vi "SR1.get Number of Stored Data.vi"(0 "i ref in":refnum<vi>, 5 "error in (no error)":errorcluster) -> (14 "i ref out":refnum<vi>, 16 "NofStoredData":i32, 19 "error out":errorcluster)   [LabVIEW 2014, in "SR1.lvlib"]
doc: "reads the number of measurements (triggers) since the last start cmd"
uses:
  SR1.lvlib
  CSlibraries/UtilityLib/UtilityLib.valueStatus.ctl
  CS_Core/CSApplicationBaseClasses/NABase/NABase.directionType.ctl
  CS_Core/CSApplicationBaseClasses/NABase/NABase.serviceType.ctl
  CS_Core/CSSystem/CoreDefs/CoreDefs.error_type.ctl
  CS_Core/CSSystem/CoreLib/CoreLib.lvlib
  CSlibraries/UtilityLib/UtilityLib.lvlib
  CS_Core/CSApplicationBaseClasses/NABase/NABase.lvlib
  instr.lib/Stanford Research SR1/Stanford Research SR1.lvlib
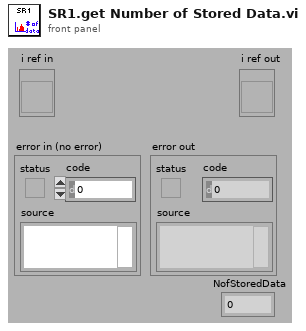
[diagram p1: front panel]
types:
  T1 = typedef "NABase.lvlib/NABase.serviceType.ctl" = enum16{"StartFreq", "NofLines", "FreqSpan", "status", "triggerLevel", "triggerSlope", "TimeRecDur", "NofStoredData"}
  T2 = typedef "NABase.lvlib/NABase.directionType.ctl" = enum16{"unknown", "update actual value", "update nominal value", "update both"}
  T3 = typedef "UtilityLib.lvlib/UtilityLib.valueStatus.ctl" = enum16{"no info available", "stand by/off", "on", "warning", "alarm/malfunction", "not implemented", "user action required", "important information", "system default", "control default", "indicator default", "button default"}
  T4 = typedef "CoreDefs.error_type.ctl" = enum16{"no error", "can't load process", "can't unload process", "process does not exist", "can't install process", "can't remove process", "unknown function", "time out", "can't execute function", "duplicate queue name", "super not found", "caller queue invalid", "can't ping process", "unknown error", "VISA Error", "VISA timeout", "GPIB timeout", "GPIB error", "communication error", "data type mismatch", "can't read data from OPC server", "can't write data to OPC server", "OET error", "function not implemented", "process already exists", "invalid Shared Variable name", "error writing Shared Variable", "error reading Shared Variable", "invalid client name", "corrupt database", "unknown class", "call not authorized", "parameter out of range", "OET timeout: can't get data to modify", "invalid queue name", "requested operation incompatible with current state", "event undefined", "event disabled", "state undefined", "caller is not a friend", "EventBuilder: bad eventID", "EventBuilder: no DAQ devices", "a thread must not stop itself", "UNUSED ELEMENT4", "DiscArchiver: eventData incomplete", "DiscArchiver: eventData does not belong to run", "DiscArchiver: can't open file", "DiscArchiver: can't write to file", "DiscArchiver: available disc space low", "can't acquire semaphore", "error reading data from database", "notifier object is not existing", "can't register process", "can't unregister process", "illegal event type", "object disabled", "object already exists", "can't change state", "Instrument not found", "no connection to remote node", "invalid reference", "N/A", "UNUSED ELEMENT 1", "element not found", "illegal TCP/IP connection detected", "object does not exist", "invalid access ID", "unknown CS system", "invalid privilige", "unsupported data type", "unsupported server type", "IO server already exists", "Shared Variable already exists"}
  T5 = typedef "SR1.lvlib/SR1.i attribute.ctl" = cluster{"GraphID":i32, "TraceID":i32}
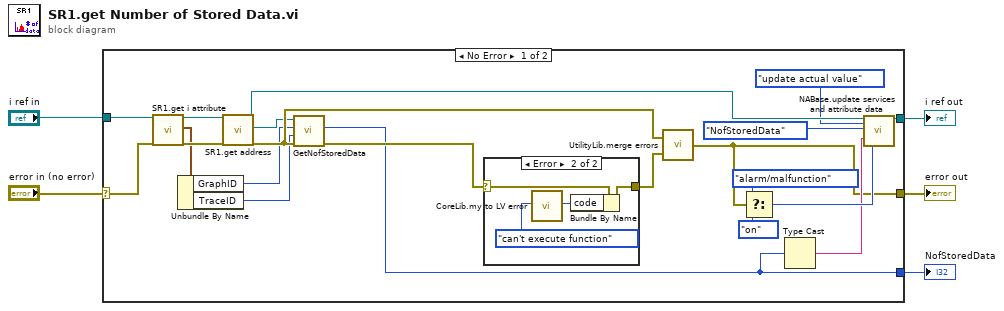
[diagram p0: block diagram]
diagram:
  n1 = case shown="No Error" "error in (no error)" {
    selector: "error in (no error)" -> [w12 w33]
    tunnel: "i ref in" -> [w10 w32]
    tunnel: [w19 w33] -> w4
    tunnel: [w20 w32] -> w3
    tunnel: [w13 _] -> w2
    frame No Error {
      n2 = call "SR1.get i attribute.vi"("i ref in"=w10, "error in (no error)"=w12) -> ("i ref out"=w9:refnum<vi>, "i attribute"=w8:T5, "error out"=w11:errorcluster)  [unwired: 15 in]
      n3 = Unbundle By Name(w8) -> ("GraphID"=w7:i32, "TraceID"=w6:i32)
      n4 = call "SR1.get address.vi"("i ref in"=w9, "error in (no error)"=w11) -> ("i ref out"=w21:refnum<vi>, "VISA resource name"=w17:refnum<visa-resource-name>, "error out"=w18:errorcluster)  [unwired: 15 in]
      n5 = call "GetNofStoredData.vi"("error in (no error)"=w18, "TraceID"=w6, "GraphID"=w7, "VISA resource name"=w17) -> ("error out"=w16:errorcluster, "StoredData"=w13:i32)  [unwired: 5 in, 1 out]
      n6 = case shown="Error" w16 {
        selector: w16 -> [w27 w31]
        tunnel: [w27 w28] -> w26
        frame No Error {
        }
        frame Error {
          n7 = call "CoreLib.my to LV error.vi"("ErrorTypes"=CoreDefs.error_type."can't execute function") -> ("LV error code"=w30:i32)  [unwired: 17 in, 1 out]
          n8 = Bundle By Name(cluster=w31, "code"=w30) -> (w28:errorcluster)
        }
      }
      n9 = call "UtilityLib.merge errors.vi"("error2 (no error)"=w26, "error1 (no error)"=w18) -> ("error out"=w19:errorcluster)
      n10 = Select(t=UtilityLib.valueStatus."alarm/malfunction" ("quality"), s=w19, f=UtilityLib.valueStatus."on") -> (s? t:f=w23:T3)
      n11 = Type Cast(x=w13) -> (*(type *) &x=w22:string)  [unwired: 1 in]
      n12 = call "NABase.update services and attribute data.vi"("i ref in"=w21, "direction"=NABase.directionType."update actual value", "service"=NABase.serviceType."NofStoredData", "value"=w22, "quality"=w23) -> ("i ref out"=w20:refnum<vi>)  [unwired: 12 in, 2 out]
    }
    frame Error {
    }
  }
  "error out" <- w4
  "i ref out" <- w3
  "NofStoredData" <- w2
